vi "读取编码器.vi"(8 "错误输入":errorcluster caption="错误输入（无错误）", 11 "设备句柄入":i32) -> (0 "错误输出":errorcluster, 1 "编码器过零值":i16[](array[numeric]), 2 "编码器AB值":i32[](array[numeric]), 3 "设备句柄":i32=1)   [LabVIEW 2016]
uses:
  dll/em9636.dll
panel:
  in  "超时毫秒":i32=1000
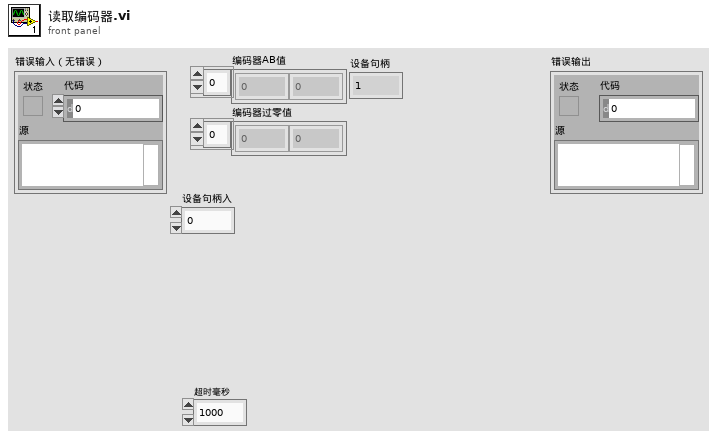
[diagram p1: front panel]
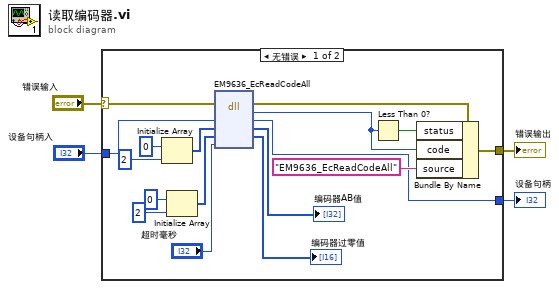
[diagram p0: block diagram]
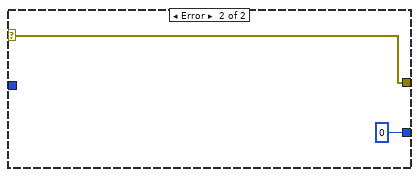
[diagram p2: hidden frame]
diagram:
  n1 = case shown="无错误" "错误输入" {
    selector: "错误输入" -> [w21 w23]
    tunnel: [w17 w23] -> w3
    tunnel: [w13 0 ("错误")] -> w2
    tunnel: "设备句柄入" -> [w15 _]
    frame No Error {
      n2 = Initialize Array(0 ("元素"), 2 ("维数大小")) -> (w11:i32[])
      n3 = Initialize Array(i16 0 ("元素"), 2 ("维数大小")) -> (w10:i16[])
      n4 = dll-call lib="PTH2kabs CUsers\nAdministratorDesktopEM9636*EM9636系列_demo_labview(调用DLL方式)dll\nem9636.dll" fn="EM9636_EcReadCodeAll"(error in=w21, "设备句柄"=w15, "abCode"=w11, "zCode"=w10, "超时毫秒"="超时毫秒") -> (error out=w19:errorcluster, "错误"=w16:i32, "设备句柄"=w13:i32, "abCode"=→"编码器AB值":i32[], "zCode"=→"编码器过零值":i16[])  [unwired: 3 in, 1 out]
      n5 = Less Than 0?(x=w16) -> (x < 0?=w18:bool)
      n6 = Bundle By Name(cluster=w19, "status"=w18, "code"=w16, "source"="EM9636_EcReadCodeAll") -> (w17:errorcluster)
    }
    frame Error {
    }
  }
  "错误输出" <- w3
  "设备句柄" <- w2
